vi "Read PdfCopy.vi"(8 "error in (no error)":errorcluster, 11 "PDF Report Class in":refnum<class "PDF Report Class.lvclass">) -> (0 "error out":errorcluster, 2 "PdfCopy":refnum<k24>, 3 "PDF Report Class out":refnum<class "PDF Report Class.lvclass">)   [LabVIEW 2019, in "PDF Report Class.lvclass"]
uses:
  <userlib>/Exaprom PDF/LV Class/PDF Report Class/PDF Report Class.lvclass
  C:/Program Files/National Instruments/LabVIEW 2019/user.lib/Exaprom PDF/DLL/itextsharp.dll
  DLL/itextsharp.dll
  <userlib>/Exaprom PDF/LV Class/PDF Report Class/PDF Report Class.lvclass/PDF Report Class.ctl
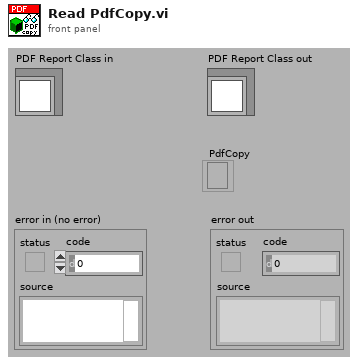
[diagram p1: front panel]
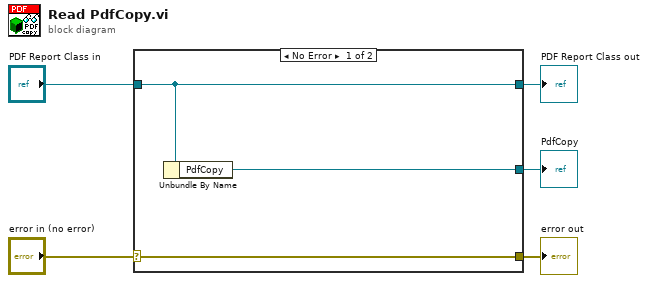
[diagram p0: block diagram]
diagram:
  n1 = case shown="No Error" "error in (no error)" {
    selector: "error in (no error)" -> [w8 w9]
    tunnel: [w8 w9] -> w4
    tunnel: [w7 w10] -> w2
    tunnel: "PDF Report Class in" -> [w7 w10]
    tunnel: [w6 _] -> w1
    frame No Error {
      n2 = Unbundle By Name(w7) -> ("PdfCopy"=w6:refnum<k24>)
    }
    frame Error {
    }
  }
  "error out" <- w4
  "PDF Report Class out" <- w2
  "PdfCopy" <- w1
